vi "getXYStage.vi"(8 "error in (no error)":errorcluster, 11 "Thorlabs APT Stage In":refnum<k7>) -> (3 "Thorlabs APT Stage Out":refnum<k7>)   [LabVIEW 2012]
uses:
  variables/GlobalUI.vi
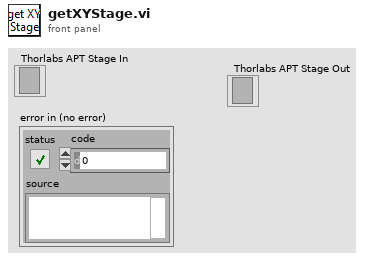
[diagram p1: front panel]
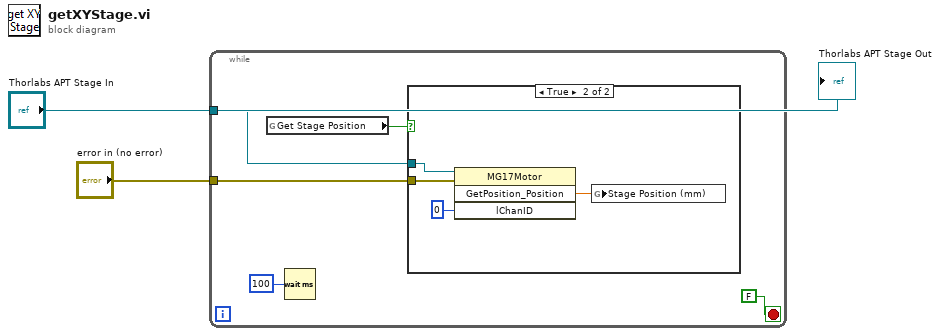
[diagram p0: block diagram]
diagram:
  n1 = while {
    tunnel: "error in (no error)" -> [w6]
    tunnel: "Thorlabs APT Stage In" -> [w4]
    stop <- FALSE stop-if-true
    n2 = global read "GlobalUI.vi" "Get Stage Position"() -> (w5:bool)
    n3 = Wait (ms)(milliseconds to wait=u32 100) -> ()  [unwired: 1 out]
    n4 = case shown="True" w5 {
      tunnel: w6 -> [_ w10]
      tunnel: w4 -> [_ w8]
      frame False {
      }
      frame True {
        n5 = invoke class="MG17Motor" method="GetPosition_Position"(reference=w8, error in=w10, "lChanID"=0) -> ("GetPosition_Position"=w9:sgl)  [unwired: 1 in, 3 out]
        n6 = global write "GlobalUI.vi" "Stage Position (mm)"(w9) -> ()
      }
    }
  }
  "Thorlabs APT Stage Out" <- "Thorlabs APT Stage In"
